vi "AlliGator Get Destination Folder.vi"(8 "Error In":errorcluster, 9 "Current Data Set (-1: single)":i32=-1, 10 "Time-Series Paths":path[](array[path]), 11 "Single Data Point Path":path) -> (0 "Error Out":errorcluster, 1 "Data Point Name":string, 3 "Destination Folder path":path)   [LabVIEW 2021, in "AlliGator Files.lvlib"]
doc: "Returns the folder in which the current dataset is saved."
uses:
  AlliGator Files.lvlib
  Files/Files.lvlib
panel:
  # "see the AlliGator License on the block diagram (Ctrl+E or Window:Show Block Diagram)"
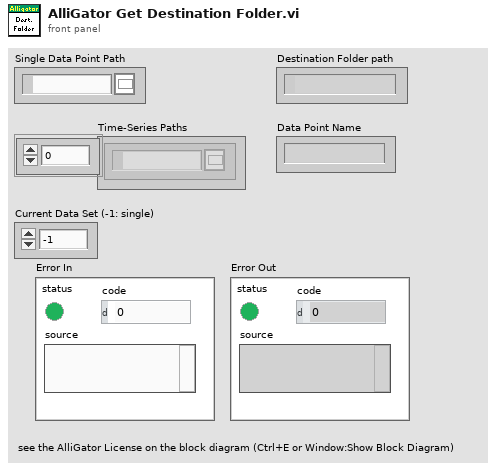
[diagram p1: front panel]
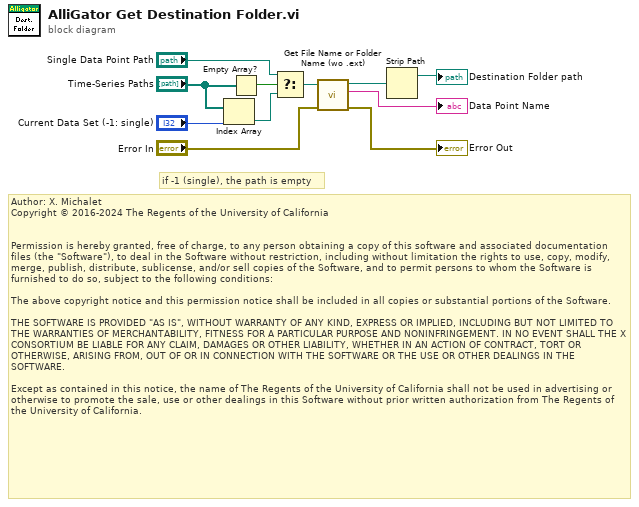
[diagram p0: block diagram]
diagram:
  # "Author: X. Michalet\nCopyright © 2016-2024 The Regents of the University of California\n \n\nPermission is hereby granted, free of charge, to any person obtaining a copy of this software and associated documentation files (the \"Software\"), to deal in the Software without restriction, including without limitation the rights to use, copy, modify, merge, publish, distribute, sublicense, and/or sell copies of the Software, and to permit persons to whom the Software is furnished to do so, subject to the following conditions:\n\nThe above copyright notice and this permission notice shall be included in all copies or substantial portions of the Software.\n\nTHE SOFTWARE IS PROVIDED \"AS IS\", WITHOUT WARRANTY OF ANY KIND, EXPRESS OR IMPLIED, INCLUDING BUT NOT LIMITED TO THE WARRANTIES OF MERCHANTABILITY, FITNESS FOR A PARTICULAR PURPOSE AND NONINFRINGEMENT. IN NO EVENT SHALL THE X CONSORTIUM BE LIABLE FOR ANY CLAIM, DAMAGES OR OTHER LIABILITY, WHETHER IN AN ACTION OF CONTRACT, TORT OR OTHERWISE, ARISING FROM, OUT OF OR IN CONNECTION WITH THE SOFTWARE OR THE USE OR OTHER DEALINGS IN THE SOFTWARE.\n\nExcept as contained in this notice, the name of The Regents of the University of California shall not be used in advertising or otherwise to promote the sale, use or other dealings in this Software without prior written authorization from The Regents of the University of California."
  # "if -1 (single), the path is empty"
  n1 = Index Array(array="Time-Series Paths", index="Current Data Set (-1: single)") -> (element=w8:path)
  n2 = Empty Array?(array="Time-Series Paths") -> (empty?=w6:bool)
  n3 = Select(t="Single Data Point Path", s=w6, f=w8) -> (s? t:f=w5:path)
  n4 = call "Get File Name or Folder Name (wo .ext).vi"("error in (no error)"="Error In", "input path"=w5) -> ("error out"=→"Error Out":errorcluster, "filename without extension"=→"Data Point Name":string, "dup path"=w4:path)  [unwired: 7 in]
  n5 = Strip Path(path=w4) -> (stripped path=→"Destination Folder path":path)  [unwired: 1 out]
